vi "CANSendMessage.vi"(8 "error in (no error)":errorcluster, 9 "Data":u8[](array[numeric]), 10 "ID":u32, 11 "CAN Cluster in":refnum<vi>) -> (0 "error out":errorcluster caption="错误输出")   [LabVIEW 2017]
uses:
  data/PCAN_Driver x64/ControlCAN.llb/VCI_CAN_OBJ.ctl
  data/PCAN_Driver x64/ControlCAN.lvlib
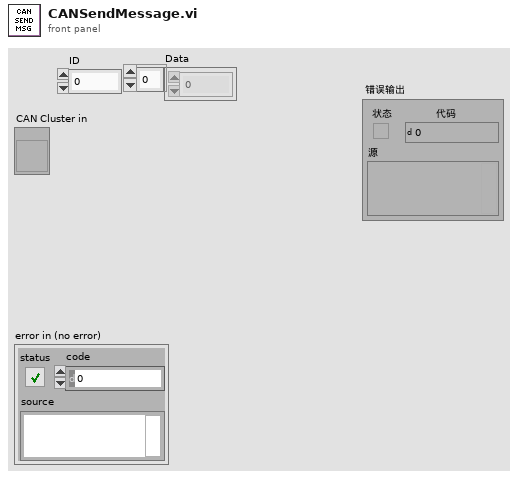
[diagram p1: front panel]
types:
  T1 = typedef "ControlCAN.lvlib/VCI_CAN_OBJ.ctl" = cluster{"ID":u32, "TimeStamp":u32, "TimeFlag":u8, "SendType":u8, "RemoteFlag":u8, "ExternFlag":u8, "DataLen":u8, "Data":u8[], "Reserved":u8[]}
  T2 = cluster{"ID":u32, "MSGTYPE":u8, "LEN":u8, "aDATA":u8[]}
  T3 = typedef "ControlCAN.lvlib/DevType.ctl" = u32
  T4 = typedef "ControlCAN.lvlib/CAN Channel.ctl" = u32
  T5 = typedef "ControlCAN.lvlib/VCI_INIT_CONFIG.ctl" = cluster{"AccCode":u32, "AccMask":u32, "InitFlag":T6, "Fliter":T7, "Timing0":u8, "Timing1":u8, "Mode":T8}
  T6 = typedef "ControlCAN.lvlib/InitFlag.ctl" = u32
  T7 = typedef "ControlCAN.lvlib/Fliter.ctl" = u8
  T8 = typedef "ControlCAN.lvlib/Mode.ctl" = u8
  T9 = cluster{"DevType":T3, "DevIndex":u32, "CanIndex":T4, "VCI_INIT_CONFIG":T5}
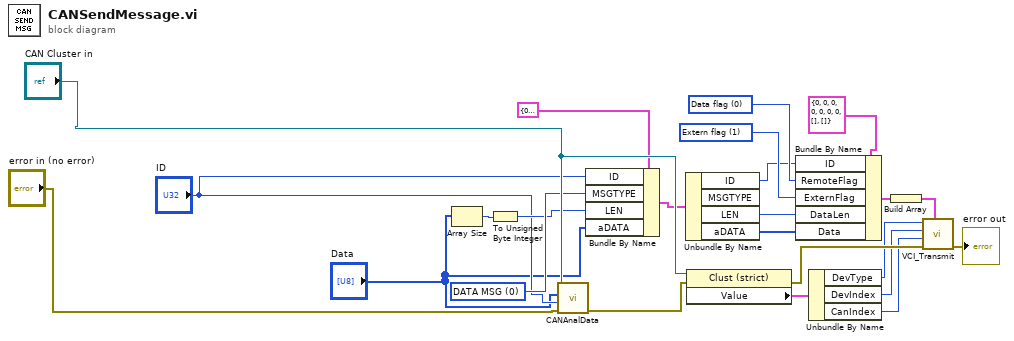
[diagram p0: block diagram]
diagram:
  w20 = u8 0 items=["STATUS"=128, "EXTENDED"=2, "RTR"=1, "DATA MSG"=0] ("MSGTYPE")
  w15 = u8 1 items=["Standart flag", "Extern flag"] ("Format")
  w16 = u8 0 items=["Data flag", "Remote flag"] ("Type")
  n1 = Array Size(array="Data") -> (size(s)=w17:i32)
  n2 = To Unsigned Byte Integer(number=w17) -> (unsigned 8bit integer=w19:u8)
  n3 = call "CANAnalData.vi"("error in"="error in (no error)", "ID"="ID", "Data"="Data", "Config"="CAN Cluster in") -> ("error out"=w24:errorcluster)  [unwired: 3 in, 4 out]
  n4 = Bundle By Name(cluster=T2 {"ID"=0, "MSGTYPE"=0, "LEN"=0, "aDATA"=[]} ("MsgTX 2"), "ID"="ID", "MSGTYPE"=w20, "LEN"=w19, "aDATA"="Data") -> (w21:T2)
  n5 = Unbundle By Name(w21) -> ("ID"=w7:u32, "LEN"=w6:u8, "aDATA"=w5:u8[])  [unwired: 1 out]
  n6 = property class="Clust (strict)"(reference="CAN Cluster in", error in=w24) -> (error out=w23:errorcluster, "Value"=w8:T9)  [unwired: 1 out]
  n7 = Bundle By Name(cluster=T1 {"ID"=0, "TimeStamp"=0, "TimeFlag"=0, "SendType"=0, "RemoteFlag"=0, "ExternFlag"=0, "DataLen"=0, "Data"=[], "Reserved"=[]} ("Send"), "ID"=w7, "RemoteFlag"=w16, "ExternFlag"=w15, "DataLen"=w6, "Data"=w5) -> (w10:T1)
  n8 = Unbundle By Name(w8) -> ("DevType"=w14:T3, "DevIndex"=w13:u32, "CanIndex"=w12:T4)
  n9 = Build Array(w10) -> (w11:T1[])
  n10 = call "VCI_Transmit.vi"("Buffer"=w11, "error in (no error)"=w23, "CANIndex"=w12, "DevIndex"=w13, "DevType"=w14) -> ("error out"=→"error out":errorcluster)  [unwired: 6 out]
